vi "fpga_LP2ControlUnit.vi"(0 "#Ch":fxp<+,5,5>=16.0, 1 "reset":bool, 2 "input valid":bool) -> (5 "ready for input":bool, 7 "output valid":bool, 8 "opState":T1, 9 "coefRDAddr":fxp<+,8,8>)   [LabVIEW 2011, in "NI_EP_PMU_FPGA.lvlib"]
uses:
  <vilib>/addons/Electrical Power/PMU/NI_EP_PMU_FPGA.lvlib
  <vilib>/rvi/FXPMathLib/basic elements/FxpAddSub/XNode/nifxpmath_AddSub.xnode
  <vilib>/rvi/FXPMathLib/sim/FxpSim.dll
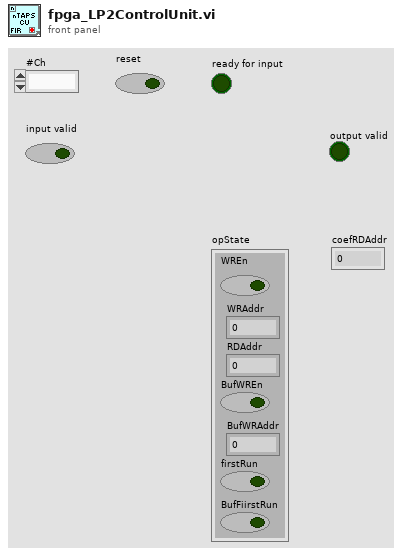
[diagram p1: front panel]
types:
  T1 = cluster{"WREn":bool, "WRAddr":fxp<+,12,12>, "RDAddr":fxp<+,12,12>, "BufWREn":bool, "BufWRAddr":fxp<+,12,12>, "firstRun":bool, "BufFiirstRun":bool}
  T2 = cluster{"idle":bool, "ready for input":bool, "macWrap":bool, "inputBufWRAddr":fxp<+,12,12>, "coefRDAddr":fxp<+,8,8>, "stateMemRDAddr":fxp<+,12,12>, "stateMemPageRDAddr":fxp<+,12,12>, "chCnt":fxp<+,5,5>, "first run?":bool, "firstRunCnt":fxp<+,12,12>, "buf first run?":bool, "bufFirstRunCnt":fxp<+,12,12>}
  T3 = cluster{"inputBufWRAddr":fxp<+,12,12>, "coefRDAddr":fxp<+,8,8>, "stateMemPageRDAddr":fxp<+,12,12>, "#Ch*#BufSize":fxp<+,12,12>, "#Ch*(#TPPM-1)-1":fxp<+,12,12>, "2*#Ch-1":fxp<+,5,5>, "#Ch*(#TPPM-2)-1":fxp<+,12,12>, "-#Ch":fxp<+,12,12>}
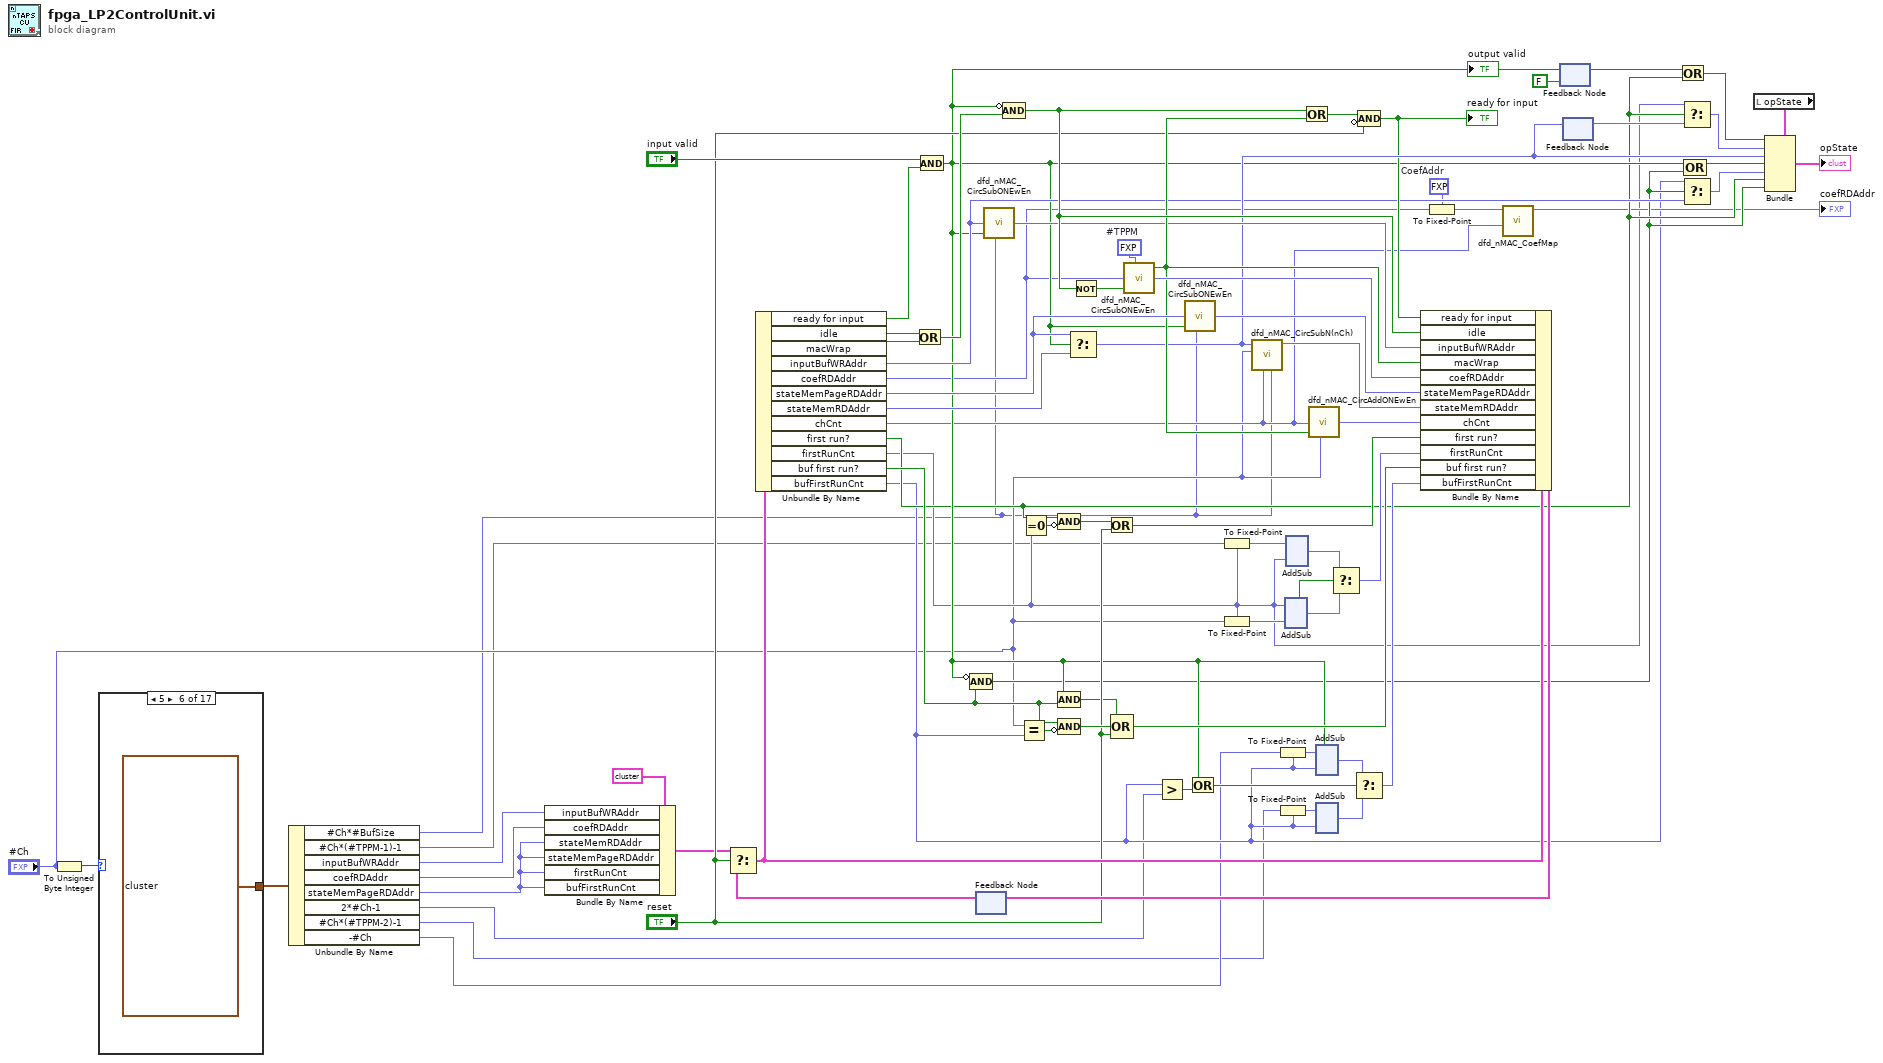
[diagram p0: block diagram]
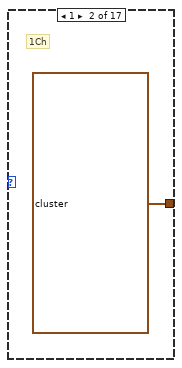
[diagram p3: hidden frame]
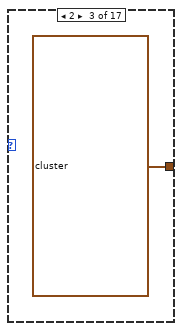
[diagram p4: hidden frame]
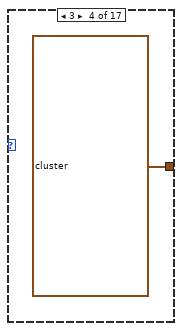
[diagram p5: hidden frame]
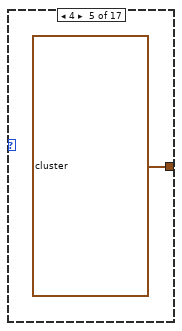
[diagram p6: hidden frame]
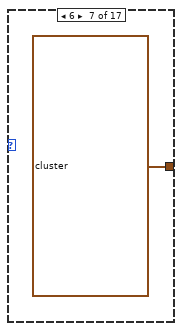
[diagram p7: hidden frame]
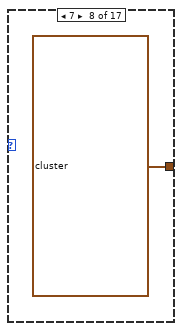
[diagram p8: hidden frame]
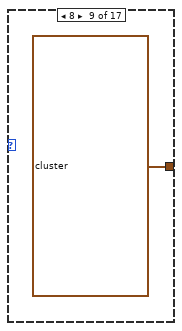
[diagram p9: hidden frame]
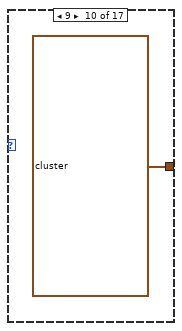
[diagram p10: hidden frame]
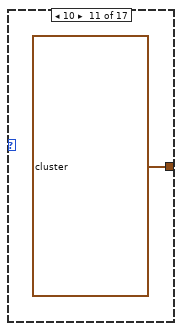
[diagram p11: hidden frame]
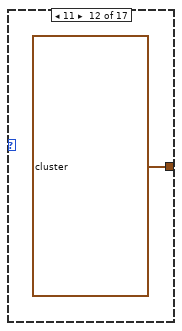
[diagram p12: hidden frame]
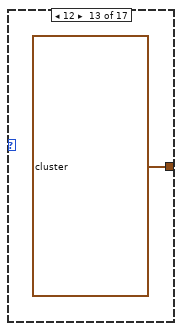
[diagram p13: hidden frame]
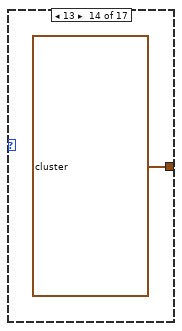
[diagram p14: hidden frame]
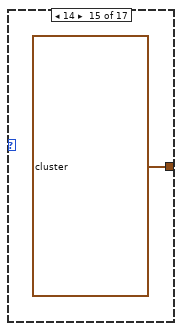
[diagram p15: hidden frame]
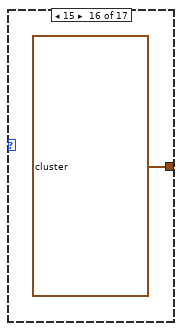
[diagram p16: hidden frame]
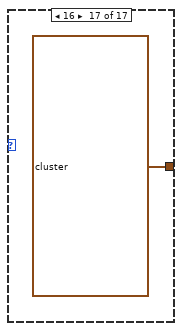
[diagram p17: hidden frame]
diagram:
  w20 = fxp<+,8,8> 0.0  # CoefAddr
  w68 = fxp<+,8,8> 213.0  # #TPPM
  n1 = To Unsigned Byte Integer(number="#Ch") -> (unsigned 8bit integer=w10:u8)
  n2 = case shown="5" w10 {
    tunnel: [_ T3 {"inputBufWRAddr"=0.0, "coefRDAddr"=212.0, "stateMemPageRDAddr"=212.0, "#Ch*#BufSize"=213.0, "#Ch*(#TPPM-1)-1"=211.0, "2*#Ch-1"=1.0, "#Ch*(#TPPM-2)-1"=210.0, "-#Ch"=4095.0} ("Cluster") T3 {"inputBufWRAddr"=1.0, "coefRDAddr"=212.0, "stateMemPageRDAddr"=425.0, "#Ch*#BufSize"=426.0, "#Ch*(#TPPM-1)-1"=423.0, "2*#Ch-1"=3.0, "#Ch*(#TPPM-2)-1"=421.0, "-#Ch"=4094.0} ("Cluster") T3 {"inputBufWRAddr"=2.0, "coefRDAddr"=212.0, "stateMemPageRDAddr"=638.0, "#Ch*#BufSize"=639.0, "#Ch*(#TPPM-1)-1"=635.0, "2*#Ch-1"=5.0, "#Ch*(#TPPM-2)-1"=632.0, "-#Ch"=4093.0} ("Cluster") T3 {"inputBufWRAddr"=3.0, "coefRDAddr"=212.0, "stateMemPageRDAddr"=851.0, "#Ch*#BufSize"=852.0, "#Ch*(#TPPM-1)-1"=847.0, "2*#Ch-1"=7.0, "#Ch*(#TPPM-2)-1"=843.0, "-#Ch"=4092.0} ("Cluster") T3 {"inputBufWRAddr"=4.0, "coefRDAddr"=212.0, "stateMemPageRDAddr"=1064.0, "#Ch*#BufSize"=1065.0, "#Ch*(#TPPM-1)-1"=1059.0, "2*#Ch-1"=9.0, "#Ch*(#TPPM-2)-1"=1054.0, "-#Ch"=4091.0} ("Cluster") T3 {"inputBufWRAddr"=5.0, "coefRDAddr"=212.0, "stateMemPageRDAddr"=1277.0, "#Ch*#BufSize"=1278.0, "#Ch*(#TPPM-1)-1"=1271.0, "2*#Ch-1"=11.0, "#Ch*(#TPPM-2)-1"=1265.0, "-#Ch"=4090.0} ("Cluster") T3 {"inputBufWRAddr"=6.0, "coefRDAddr"=212.0, "stateMemPageRDAddr"=1490.0, "#Ch*#BufSize"=1491.0, "#Ch*(#TPPM-1)-1"=1483.0, "2*#Ch-1"=13.0, "#Ch*(#TPPM-2)-1"=1476.0, "-#Ch"=4089.0} ("Cluster") T3 {"inputBufWRAddr"=7.0, "coefRDAddr"=212.0, "stateMemPageRDAddr"=1703.0, "#Ch*#BufSize"=1704.0, "#Ch*(#TPPM-1)-1"=1695.0, "2*#Ch-1"=15.0, "#Ch*(#TPPM-2)-1"=1687.0, "-#Ch"=4088.0} ("Cluster") T3 {"inputBufWRAddr"=8.0, "coefRDAddr"=212.0, "stateMemPageRDAddr"=1916.0, "#Ch*#BufSize"=1917.0, "#Ch*(#TPPM-1)-1"=1907.0, "2*#Ch-1"=17.0, "#Ch*(#TPPM-2)-1"=1898.0, "-#Ch"=4087.0} ("Cluster") T3 {"inputBufWRAddr"=9.0, "coefRDAddr"=212.0, "stateMemPageRDAddr"=2129.0, "#Ch*#BufSize"=2130.0, "#Ch*(#TPPM-1)-1"=2119.0, "2*#Ch-1"=19.0, "#Ch*(#TPPM-2)-1"=2109.0, "-#Ch"=4086.0} ("Cluster") T3 {"inputBufWRAddr"=10.0, "coefRDAddr"=212.0, "stateMemPageRDAddr"=2342.0, "#Ch*#BufSize"=2343.0, "#Ch*(#TPPM-1)-1"=2331.0, "2*#Ch-1"=21.0, "#Ch*(#TPPM-2)-1"=2320.0, "-#Ch"=4085.0} ("Cluster") T3 {"inputBufWRAddr"=11.0, "coefRDAddr"=212.0, "stateMemPageRDAddr"=2555.0, "#Ch*#BufSize"=2556.0, "#Ch*(#TPPM-1)-1"=2543.0, "2*#Ch-1"=23.0, "#Ch*(#TPPM-2)-1"=2531.0, "-#Ch"=4084.0} ("Cluster") T3 {"inputBufWRAddr"=12.0, "coefRDAddr"=212.0, "stateMemPageRDAddr"=2768.0, "#Ch*#BufSize"=2769.0, "#Ch*(#TPPM-1)-1"=2755.0, "2*#Ch-1"=25.0, "#Ch*(#TPPM-2)-1"=2742.0, "-#Ch"=4083.0} ("Cluster") T3 {"inputBufWRAddr"=13.0, "coefRDAddr"=212.0, "stateMemPageRDAddr"=2981.0, "#Ch*#BufSize"=2982.0, "#Ch*(#TPPM-1)-1"=2967.0, "2*#Ch-1"=27.0, "#Ch*(#TPPM-2)-1"=2953.0, "-#Ch"=4082.0} ("Cluster") T3 {"inputBufWRAddr"=14.0, "coefRDAddr"=212.0, "stateMemPageRDAddr"=3194.0, "#Ch*#BufSize"=3195.0, "#Ch*(#TPPM-1)-1"=3179.0, "2*#Ch-1"=29.0, "#Ch*(#TPPM-2)-1"=3164.0, "-#Ch"=4081.0} ("Cluster") T3 {"inputBufWRAddr"=15.0, "coefRDAddr"=212.0, "stateMemPageRDAddr"=3407.0, "#Ch*#BufSize"=3408.0, "#Ch*(#TPPM-1)-1"=3391.0, "2*#Ch-1"=31.0, "#Ch*(#TPPM-2)-1"=3375.0, "-#Ch"=4080.0} ("Cluster")] -> w9
    frame 0, Default {
    }
    frame 1 {
      # "1Ch"
    }
    frame 2 {
    }
    frame 3 {
    }
    frame 4 {
    }
    frame 5 {
    }
    frame 6 {
    }
    frame 7 {
    }
    frame 8 {
    }
    frame 9 {
    }
    frame 10 {
    }
    frame 11 {
    }
    frame 12 {
    }
    frame 13 {
    }
    frame 14 {
    }
    frame 15 {
    }
    frame 16 {
    }
  }
  n3 = Unbundle By Name(w9) -> ("#Ch*#BufSize"=w1:fxp<+,12,12>, "#Ch*(#TPPM-1)-1"=w2:fxp<+,12,12>, "inputBufWRAddr"=w3:fxp<+,12,12>, "coefRDAddr"=w4:fxp<+,8,8>, "stateMemPageRDAddr"=w5:fxp<+,12,12>, "2*#Ch-1"=w6:fxp<+,5,5>, "#Ch*(#TPPM-2)-1"=w7:fxp<+,12,12>, "-#Ch"=w8:fxp<+,12,12>)
  n4 = Bundle By Name(cluster=T2 {"idle"=TRUE, "ready for input"=FALSE, "macWrap"=FALSE, "inputBufWRAddr"=15.0, "coefRDAddr"=212.0, "stateMemRDAddr"=3407.0, "stateMemPageRDAddr"=3407.0, "chCnt"=0.0, "first run?"=TRUE, "firstRunCnt"=3407.0, "buf first run?"=TRUE, "bufFirstRunCnt"=3407.0} ("CUInitialState"), "inputBufWRAddr"=w3, "coefRDAddr"=w4, "stateMemRDAddr"=w5, "stateMemPageRDAddr"=w5, "firstRunCnt"=w5, "bufFirstRunCnt"=w5) -> (w12:T2)
  n5 = feedback #1() -> (w69:T2)  [unwired: 1 out]
  n6 = Select(t=w12, s="reset", f=w69) -> (s? t:f=w66:T2)
  n7 = Unbundle By Name(w66) -> ("ready for input"=w64:bool, "idle"=w56:bool, "macWrap"=w57:bool, "inputBufWRAddr"=w43:fxp<+,12,12>, "coefRDAddr"=w21:fxp<+,8,8>, "stateMemPageRDAddr"=w72:fxp<+,12,12>, "stateMemRDAddr"=w73:fxp<+,12,12>, "chCnt"=w23:fxp<+,5,5>, "first run?"=w26:bool, "firstRunCnt"=w17:fxp<+,12,12>, "buf first run?"=w29:bool, "bufFirstRunCnt"=w14:fxp<+,12,12>)
  n8 = Or(x=w56, y=w57) -> (x .or. y?=w63:bool)
  n9 = And(x="input valid", y=w64) -> (x .and. y?=w28:bool)
  "output valid" <- w28
  n10 = Compound Arithmetic op=AND(invert w28, w29) -> (w25:bool)
  n11 = call "dfd_nMAC_CircSubONEwEn.vi"("len"=w1, "idxIn"=w43, "Enable"=w28) -> ("idxOut"=w59:fxp<+,12,12>)  [unwired: 5 in, 1 out]
  n12 = Compound Arithmetic op=AND(invert w28, w63) -> (w62:bool)
  n13 = Equal?(x="#Ch", y=w14) -> (x = y?=w54:bool)
  n14 = Equal To 0?(x=w17) -> (x = 0?=w38:bool)
  n15 = Compound Arithmetic op=AND(w26, invert w38) -> (w39:bool)
  n16 = Compound Arithmetic op=AND(w28, w29) -> (w27:bool)
  n17 = Compound Arithmetic op=AND(w29, invert w54) -> (w53:bool)
  n18 = Select(t=w72, s=w28, f=w73) -> (s? t:f=w58:fxp<+,12,12>)
  n19 = Not(x=w62) -> (.not. x?=w70:bool)
  n20 = Or(x=w39, y="reset") -> (x .or. y?=w35:bool)
  n21 = Compound Arithmetic op=OR(w27, w53, "reset") -> (w33:bool)
  n22 = call "dfd_nMAC_CircSubONEwEn.vi"("len"=w68, "idxIn"=w21, "Enable"=w70) -> ("wrap?"=w60:bool, "idxOut"=w75:fxp<+,8,8>)  [unwired: 5 in]
  n23 = Greater?(x=w14, y=w6) -> (0:w37:bool)
  n24 = call "dfd_nMAC_CircSubONEwEn.vi"("len"=w1, "idxIn"=w72, "Enable"=w28) -> ("idxOut"=w74:fxp<+,12,12>)  [unwired: 5 in, 1 out]
  n25 = Or(x=w28, y=w37) -> (x .or. y?=w36:bool)
  n26 = To Fixed-Point(fixed-point type=w17, number=w2) -> (fixed-point=w19:fxp<+,12,12>)
  n27 = To Fixed-Point(fixed-point type=w17, number="#Ch") -> (fixed-point=w18:fxp<+,12,12>)
  n28 = call "dfd_nMAC_CircSubN(nCh).vi"("bufSize*#ch"=w1, "curChIdx"=w23, "#ch"="#Ch", "idxIn"=w58) -> ("idxOut"=w77:fxp<+,12,12>)  [unwired: 7 in]
  n29 = To Fixed-Point(fixed-point type=w14, number=w8) -> (fixed-point=w16:fxp<+,12,12>)
  n30 = To Fixed-Point(fixed-point type=w14, number=w7) -> (fixed-point=w15:fxp<+,12,12>)
  n31 = xnode ("AddSub")("x"=w17, "y"=w18) -> ("s"=w42:fxp<+,12,12>, "borrow-out"=w41:bool)
  n32 = xnode ("AddSub")("x"=w19, "y"=w17) -> ("s"=w40:fxp<+,12,12>)  [unwired: 1 out]
  n33 = Or(x=w62, y=w60) -> (x .or. y?=w61:bool)
  n34 = call "dfd_nMAC_CircAddONEwEn.vi"("len"="#Ch", "idxIn"=w23, "Enable"=w60) -> ("idxOut"=w76:fxp<+,5,5>)  [unwired: 5 in, 1 out]
  n35 = xnode ("AddSub")("x"=w16, "y"=w14, "use zero instead of x"=w28) -> ("s"=w50:fxp<+,12,12>)  [unwired: 1 out]
  n36 = xnode ("AddSub")("x"=w15, "y"=w14) -> ("s"=w51:fxp<+,12,12>)  [unwired: 1 out]
  n37 = Select(t=w40, s=w41, f=w42) -> (s? t:f=w34:fxp<+,12,12>)
  n38 = Select(t=w50, s=w36, f=w51) -> (s? t:f=w32:fxp<+,12,12>)
  n39 = Compound Arithmetic op=AND(w61, invert "reset") -> (w55:bool)
  "ready for input" <- w55
  n40 = Bundle By Name(cluster=w66, "ready for input"=w55, "idle"=w62, "inputBufWRAddr"=w59, "macWrap"=w60, "coefRDAddr"=w75, "stateMemPageRDAddr"=w74, "stateMemRDAddr"=w77, "chCnt"=w76, "first run?"=w35, "firstRunCnt"=w34, "buf first run?"=w33, "bufFirstRunCnt"=w32) -> (w67:T2)
  n41 = feedback-in #1(w67) -> ()
  n42 = To Fixed-Point(fixed-point type=w20, number=w21) -> (fixed-point=w22:fxp<+,8,8>)
  n43 = call "dfd_nMAC_CoefMap.vi"("chCnt"=w23, "coefOffsetAddr"=w22) -> ("coefRDAddr"=→"coefRDAddr":fxp<+,8,8>)  [unwired: 9 in]
  n44 = feedback-in #2(w28) -> ()
  n45 = feedback #2(FALSE) -> (w49:bool)
  n46 = feedback-in #3(w58) -> ()
  n47 = feedback #3() -> (w47:fxp<+,12,12>)  [unwired: 1 out]
  n48 = Or(x=w49, y=w26) -> (x .or. y?=w48:bool)
  n49 = Select(t=w17, s=w26, f=w47) -> (s? t:f=w46:fxp<+,12,12>)
  n50 = Select(t=w14, s=w25, f=w43) -> (s? t:f=w45:fxp<+,12,12>)
  n51 = Compound Arithmetic op=OR(w28, w25) -> (w44:bool)
  n52 = local read "opState"() -> (w30:T1)
  n53 = Bundle(cluster=w30, "WREn"=w48, "WRAddr"=w46, "RDAddr"=w58, "BufWREn"=w44, "BufWRAddr"=w45, "firstRun"=w26, "BufFiirstRun"=w25) -> (→"opState":T1)
